vi "Write Exception list and Save all mode.vi"(8 "error in (no error)":errorcluster, 9 "Store all mode?(T)":bool=TRUE, 10 "Exception list":string[](array[string]), 11 "Data Repository in":refnum<class "Data Repository.lvclass">) -> (0 "error out":errorcluster, 3 "Data Repository out":refnum<class "Data Repository.lvclass">)   [LabVIEW 2020, in "Data Repository.lvlib" / "Data Repository.lvclass"]
doc: "Write exeption list and store all boolean to the class data."
uses:
  Data Repository.lvclass
  Data Repository.lvclass/Data Repository.ctl
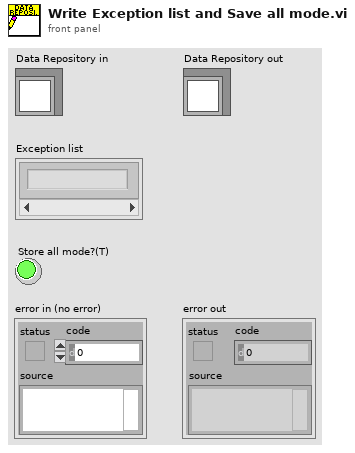
[diagram p1: front panel]
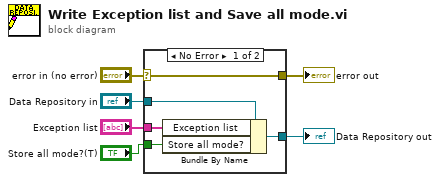
[diagram p0: block diagram]
diagram:
  n1 = case shown="No Error" "error in (no error)" {
    selector: "error in (no error)" -> [w11 w12]
    tunnel: [w11 w12] -> w5
    tunnel: [w9 w13] -> w3
    tunnel: "Data Repository in" -> [w10 w13]
    tunnel: "Exception list" -> [w8 _]
    tunnel: "Store all mode?(T)" -> [w7 _]
    frame No Error {
      n2 = Bundle By Name(cluster=w10, "Exception list"=w8, "Store all mode?"=w7) -> (w9:refnum<class "Data Repository.lvclass">)
    }
    frame Error {
    }
  }
  "error out" <- w5
  "Data Repository out" <- w3
